vi "New Queue.vi"(9 "Depth":i32, 11 "Channel Data In":T1) -> (1 "Queue":refnum<queue>, 3 "Channel Data":T1)   [LabVIEW 2020, in "Flex.lvlib"]
uses:
  Flex.lvlib
  Channel Data.ctl
  Element Info.ctl
  Event Data.ctl
  Element.ctl
  Queue Data.ctl
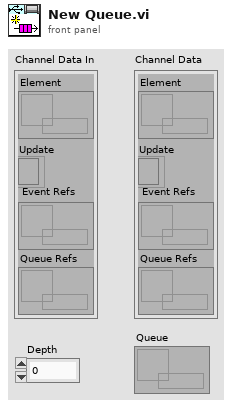
[diagram p1: front panel]
types:
  T1 = typedef "Flex.lvlib/Channel Data.ctl" = cluster{"Element":refnum<data-value>, "Update":refnum<k4>, "Event Refs":refnum<data-value>, "Queue Refs":refnum<data-value>}
  T2 = typedef "Flex.lvlib/Queue Data.ctl" = cluster{"element":T3, "Flags":u8}
  T3 = typedef "Flex.lvlib/Element.ctl" = dbl
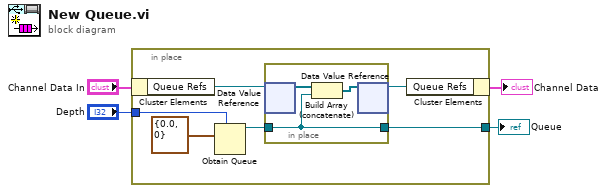
[diagram p0: block diagram]
diagram:
  n1 = in-place {
    in-place-border: "Depth" -> [w8]
    in-place-border: [w6] -> w1
    n2 = in-place-cluster #1("Channel Data In") -> ("Queue Refs"=w10:refnum<data-value>)
    n3 = Obtain Queue(max queue size (-1, unlimited)=w8, element data type=T2 {"element"=0.0, "Flags"=0} ("Queue Data")) -> (queue out=w7:refnum<queue>)  [unwired: 3 in, 2 out]
    n4 = in-place {
      in-place-border: w7 -> [w11]
      in-place-border: [w11] -> w6
      n5 = in-place-dvr #2(w10) -> (w13:refnum<queue>[])  [unwired: 1 out]
      n6 = Build Array (concatenate)(w13, w11) -> (w12:refnum<queue>[])
      n7 = in-place-dvr #2(w12) -> (w9:refnum<data-value>)  [unwired: 1 out]
    }
    n8 = in-place-cluster #1("Queue Refs"=w9) -> (→"Channel Data":T1)
  }
  "Queue" <- w1
